vi "Periods (subVI).vi"(2 "Period (usec)":u32, 3 "Duty Cycle":fxp<+/-,64,12> format="%.56g") -> (0 "High Period (us)":u32, 1 "Low Period (us)":u32)   [LabVIEW 2016]
doc: "This subVI supports a PWM output application. It translates a period and duty cycle into respective high and low periods to output via PWM."
panel:
  # "This subVI supports a PWM output application.  It translates a period and duty cycle into respective high and low periods to output via PWM."
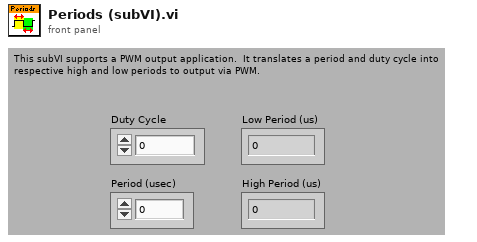
[diagram p1: front panel]
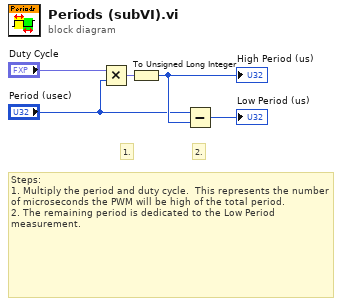
[diagram p0: block diagram]
diagram:
  # "2."
  # "1."
  # "Steps:\n1. Multiply the period and duty cycle.  This represents the number of microseconds the PWM will be high of the total period.\n2. The remaining period is dedicated to the Low Period measurement."
  n1 = Multiply(x="Duty Cycle", y="Period (usec)") -> (x*y=w4:fxp<+/-,64,43>)
  n2 = To Unsigned Long Integer(number=w4) -> (unsigned 32bit integer=w3:u32)
  "High Period (us)" <- w3
  n3 = Subtract(x="Period (usec)", y=w3) -> (x-y=→"Low Period (us)":u32)
